vi "Read.vi"(8 "error in (no error)":errorcluster, 9 "timeout ms (5000)":i32=5000, 11 "WebSocket Connection in":refnum<k5>) -> (0 "error out":errorcluster, 1 "Opcode out":T1, 2 "Data":string, 3 "WebSocket Connection out":refnum<k5>)   [LabVIEW 2017, in "LV WebSockets.lvlib"]
doc: "Reads and decodes an incoming WebSockets message.\nWebSockets 1.6.0.22\nSam Sharp - MediaMongrels Ltd\nCopyright (c) 2016, MediaMongrels Ltd"
uses:
  LV WebSockets.lvlib
  Opcode.ctl
panel:
  out "Final Frame Bit":bool
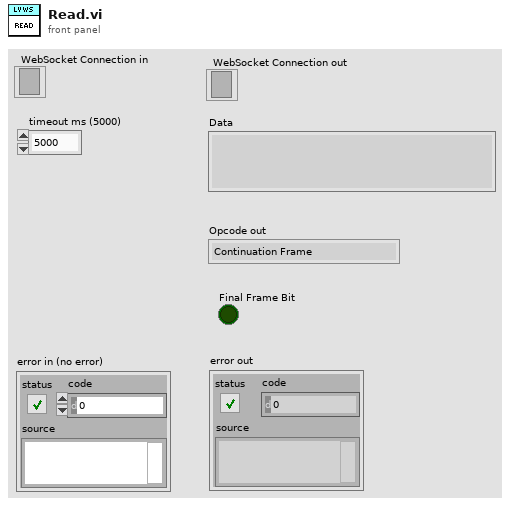
[diagram p1: front panel]
types:
  T1 = typedef "LV WebSockets.lvlib/Opcode.ctl" = enum8{"Continuation Frame", "Text Frame", "Binary Frame", "Reserved 3", "Reserved 4", "Reserved 5", "Reserved 6", "Reserved 7", "Connection Close", "Ping", "Pong", "Reserved B", "Reserved C", "Reserved D", "Reserved F"}
  T2 = enum16{"big-endian, network order", "native, host order", "little-endian"}
  T3 = enum16{"Standard", "Buffered", "CRLF", "Immediate"}
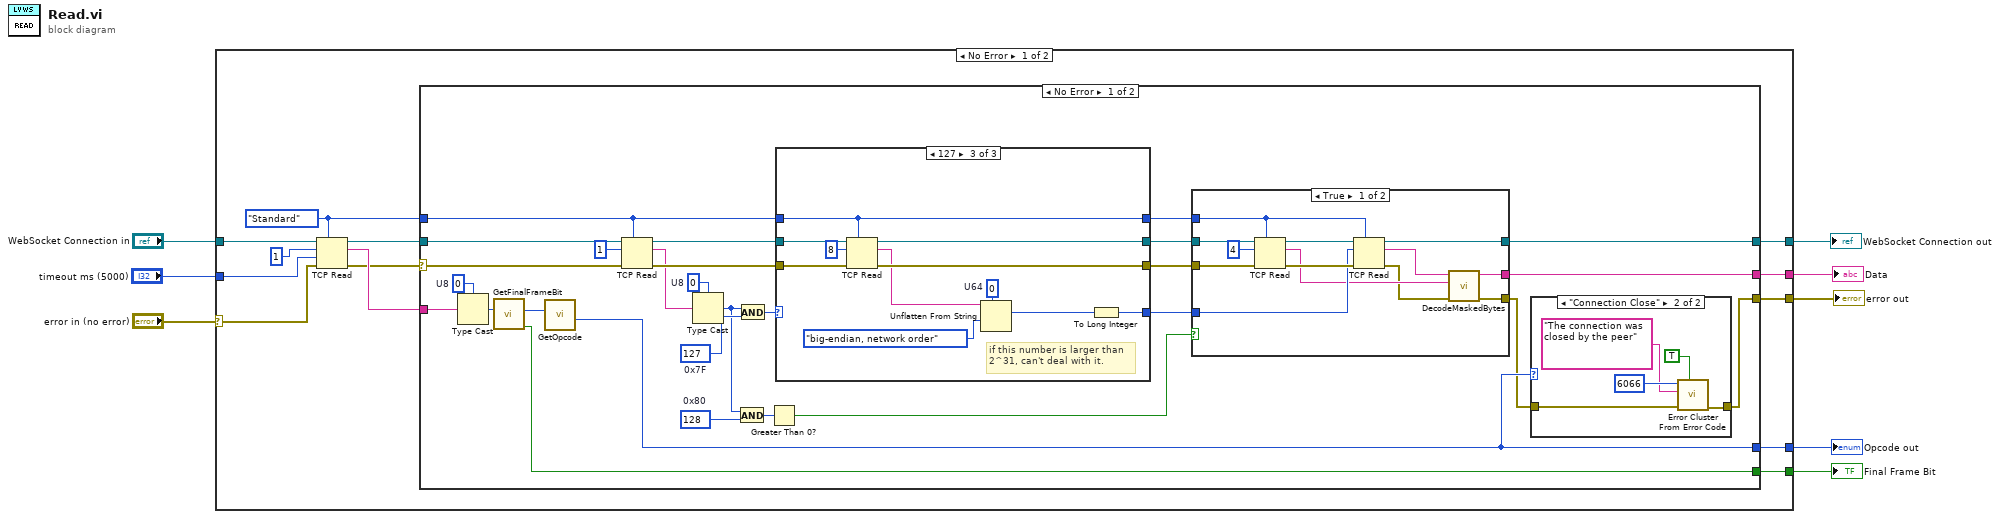
[diagram p0: block diagram]
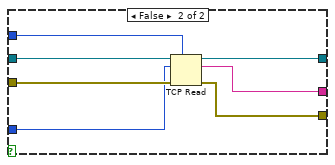
[diagram p3: hidden frame]
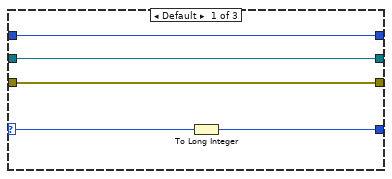
[diagram p4: hidden frame]
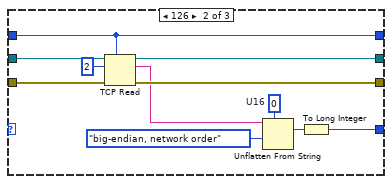
[diagram p5: hidden frame]
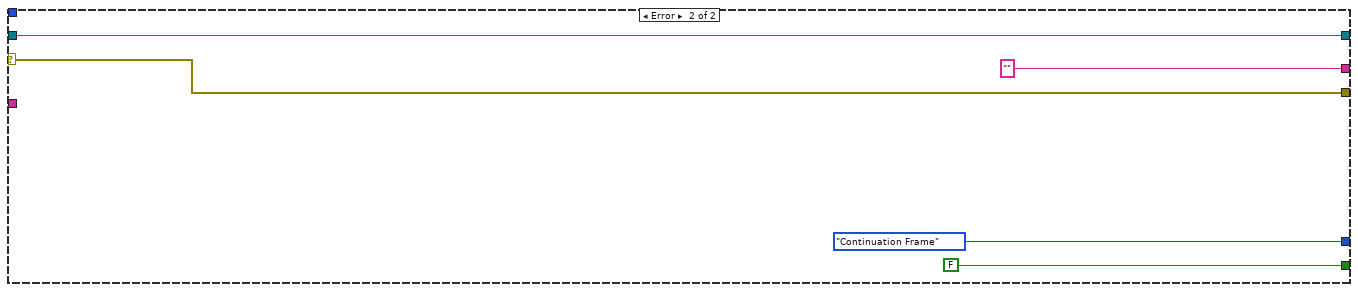
[diagram p6: hidden frame]
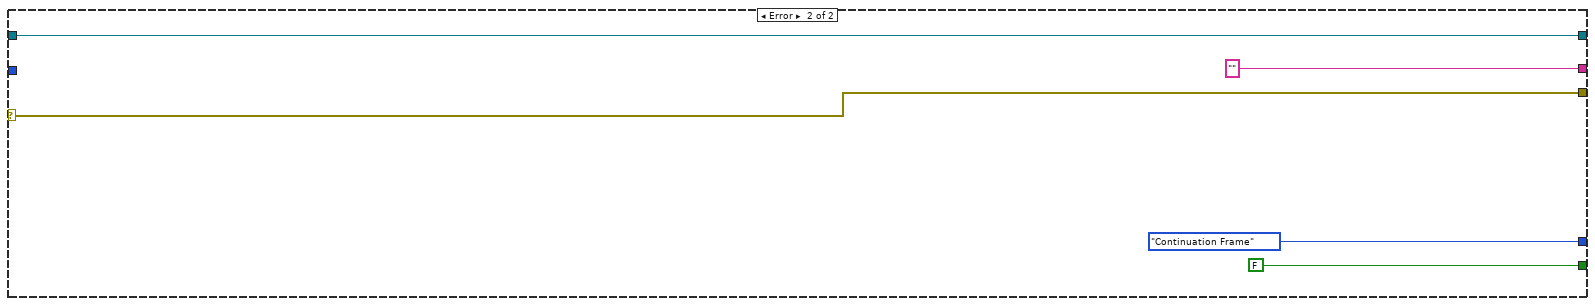
[diagram p7: hidden frame]
diagram:
  n1 = case shown="No Error" "error in (no error)" {
    selector: "error in (no error)" -> [w15 w112]
    tunnel: "WebSocket Connection in" -> [w21 w111]
    tunnel: [w16 w111] -> w7
    tunnel: [w14 "" ("data out")] -> w6
    tunnel: [w13 w112] -> w4
    tunnel: "timeout ms (5000)" -> [w12 _]
    tunnel: [w10 Opcode."Continuation Frame"] -> w2
    tunnel: [w9 FALSE ("Final Frame Bit")] -> w1
    frame No Error {
      w17 = T3."Standard" ("mode (standard)")
      n2 = TCP Read(connection ID=w21, bytes to read=1, error in (no error)=w15, 7:w17, 9:w12) -> (connection ID out=w18:refnum<k5>, data out=w19:string, error out=w11:errorcluster)
      n3 = case shown="No Error" w11 {
        selector: w11 -> [w45 w105]
        tunnel: w19 -> [w44 _]
        tunnel: w18 -> [w49 w107]
        tunnel: w17 -> [w48 _]
        tunnel: [w47 w107] -> w16
        tunnel: [w46 "" ("Decoded Data")] -> w14
        tunnel: [w22 w105] -> w13
        tunnel: [w24 Opcode."Continuation Frame"] -> w10
        tunnel: [w41 FALSE ("Final Frame Bit")] -> w9
        frame No Error {
          w29 = u8 128  # 0x80
          w30 = u8 0  # U8
          w40 = u8 127  # 0x7F
          w43 = u8 0  # U8
          n4 = Type Cast(type=w43, x=w44) -> (*(type *) &x=w42:u8)
          n5 = call "GetFinalFrameBit.vi"("Byte Packet"=w42) -> ("Final Frame Bit"=w41:bool, "Byte Packet out"=w25:u8)  [unwired: 8 in]
          n6 = call "GetOpcode.vi"("Byte Packet in"=w25) -> ("Opcode"=w24:T1)  [unwired: 8 in, 1 out]
          n7 = TCP Read(connection ID=w49, bytes to read=1, error in (no error)=w45, 7:w48) -> (connection ID out=w34:refnum<k5>, data out=w31:string, error out=w32:errorcluster)  [unwired: 1 in]
          n8 = Type Cast(type=w30, x=w31) -> (*(type *) &x=w28:u8)
          n9 = And(x=w28, y=w29) -> (x .and. y?=w27:u8)
          n10 = And(x=w28, y=w40) -> (x .and. y?=w39:u8)
          n11 = Greater Than 0?(x=w27) -> (x > 0?=w26:bool)
          n12 = case shown="127" w39 {
            selector: w39 -> [w79 _ _]
            tunnel: w34 -> [w80 w91 w101]
            tunnel: [w80 w90 w100] -> w38
            tunnel: w48 -> [w77 w88 w96]
            tunnel: [w78 w81 w99] -> w35
            tunnel: [w77 w88 w96] -> w37
            tunnel: [w76 w87 w98] -> w36
            tunnel: w32 -> [w76 w86 w97]
            frame Default {
              n13 = To Long Integer(number=w79) -> (32bit integer=w78:i32)
            }
            frame 126 {
              w85 = u16 0  # U16
              n14 = TCP Read(connection ID=w91, bytes to read=2, error in (no error)=w86, 7:w88) -> (connection ID out=w90:refnum<k5>, data out=w83:string, error out=w87:errorcluster)  [unwired: 1 in]
              n15 = Unflatten From String(type=w85, binary string=w83, byte order (0:big-endian, network order)=T2."big-endian, network order") -> (value=w82:u16)  [unwired: 2 in, 2 out]
              n16 = To Long Integer(number=w82) -> (32bit integer=w81:i32)
            }
            frame 127 {
              w95 = u64 0  # U64
              # "if this number is larger than\n2^31, can't deal with it."
              n17 = TCP Read(connection ID=w101, bytes to read=8, error in (no error)=w97, 7:w96) -> (connection ID out=w100:refnum<k5>, data out=w94:string, error out=w98:errorcluster)  [unwired: 1 in]
              n18 = Unflatten From String(type=w95, binary string=w94, byte order (0:big-endian, network order)=T2."big-endian, network order") -> (value=w93:u64)  [unwired: 2 in, 2 out]
              n19 = To Long Integer(number=w93) -> (32bit integer=w99:i32)
            }
          }
          n20 = case shown="True" w26 {
            tunnel: [w68 w75] -> w47
            tunnel: w38 -> [w67 w74]
            tunnel: w37 -> [w65 w73]
            tunnel: w36 -> [w64 w72]
            tunnel: w35 -> [w61 w71]
            tunnel: [w58 w69] -> w46
            tunnel: [w56 w70] -> w23
            frame True {
              n21 = TCP Read(connection ID=w67, bytes to read=4, error in (no error)=w64, 7:w65) -> (connection ID out=w66:refnum<k5>, data out=w60:string, error out=w63:errorcluster)  [unwired: 1 in]
              n22 = TCP Read(connection ID=w66, bytes to read=w61, error in (no error)=w63, 7:w65) -> (connection ID out=w68:refnum<k5>, data out=w59:string, error out=w57:errorcluster)  [unwired: 1 in]
              n23 = call "DecodeMaskedBytes.vi"("error in (no error)"=w57, "Mask Bytes"=w60, "Encoded Data"=w59) -> ("error out"=w56:errorcluster, "Decoded Data"=w58:string)  [unwired: 7 in]
            }
            frame False {
              n24 = TCP Read(connection ID=w74, bytes to read=w71, error in (no error)=w72, 7:w73) -> (connection ID out=w75:refnum<k5>, data out=w69:string, error out=w70:errorcluster)  [unwired: 1 in]
            }
          }
          n25 = case shown="\"Connection Close\"" w24 {
            tunnel: w23 -> [w50 w55]
            tunnel: [w50 w54] -> w22
            frame Default {
            }
            frame "Connection Close" {
              n26 = call <vilib>:"Error Cluster From Error Code.vi"("show call chain? (False)"=TRUE, "error in (no error)"=w55, "error message (\"\")"="The connection was closed by the peer" ("error message (\"\")"), "error code (0)"=6066) -> ("error out"=w54:errorcluster)  [unwired: 5 in]
            }
          }
        }
        frame Error {
        }
      }
    }
    frame Error {
    }
  }
  "WebSocket Connection out" <- w7
  "Data" <- w6
  "error out" <- w4
  "Opcode out" <- w2
  "Final Frame Bit" <- w1
